vi "Test Depth.vi"() -> ()   [LabVIEW 2017]
doc: "Using the colors from the graph, make lines radiate from robot center in the direction of the camera. Depth values of 0 and maxInt are turned into NaNs, and that is the returned line of values."
uses:
  <vilib>/addons/RealSense/libRealSense3.lvlib
  <vilib>/Analysis/NI_AALPro.lvlib
  <vilib>/Analysis/NI_AALBase.lvlib
  <vilib>/vision/NI_Vision_Development_Module.lvlib
panel:
  in  "point offset":i32=15
  out "Array":T1(array[cluster])
  in  "side points":i32=15
  in  "Line #":i32(slide) scale=1.0..10.0
  out "Formula":string
  out "error":i32
  in  "Dialate":bool
  in  "File":bool
  in  "File #":i32(slide) scale=1.0..10.0
  out "Slope":dbl[][](graph)
  in  "Lines":i32=10
  out "Friltered":cluster{i32[], dbl[]}(graph)
  out "Image":T2(plugin-control)
  out "error out":errorcluster
  in  "stop":bool
  out "device count":i32
  # "All errors are #1, string is good"
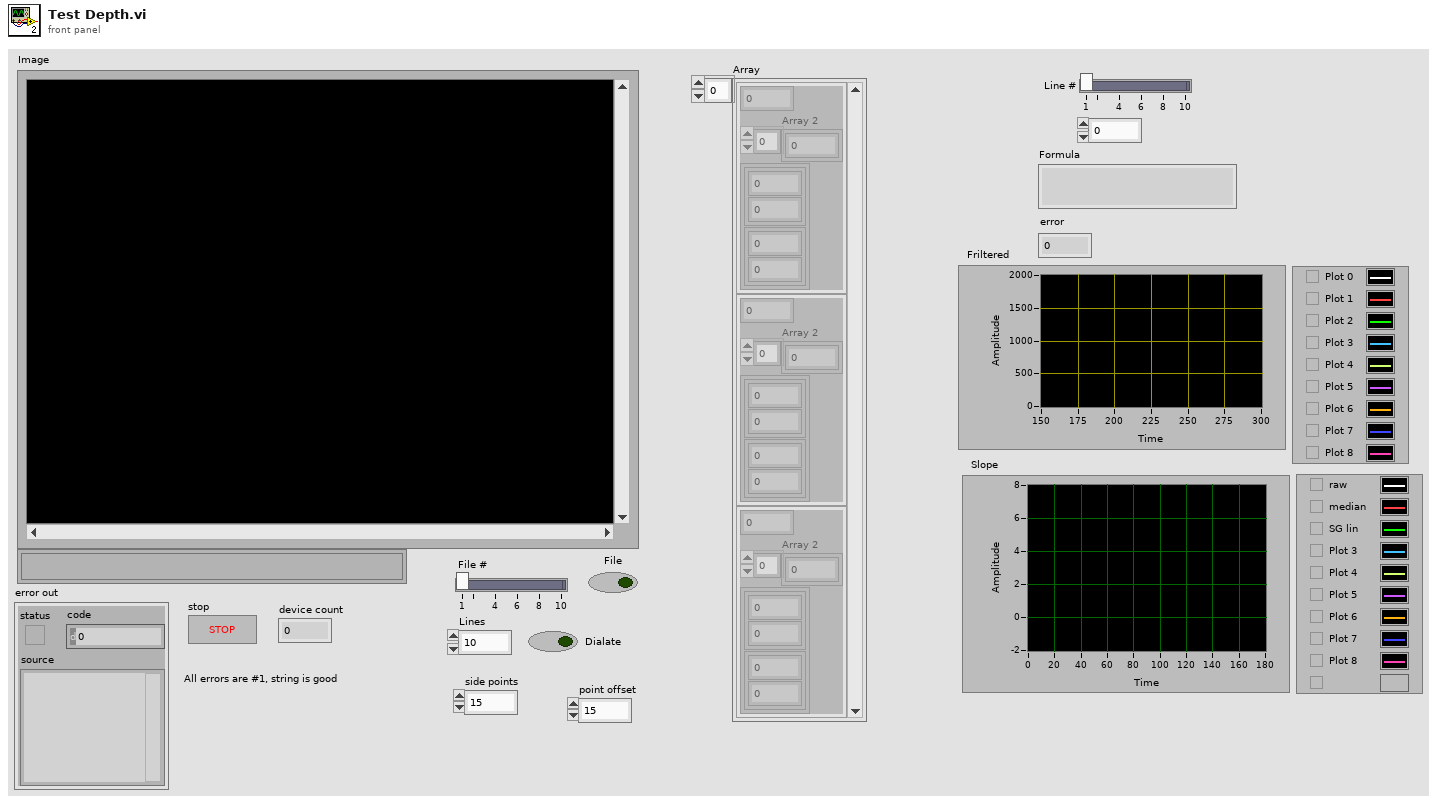
[diagram p1: front panel]
types:
  T1 = cluster{i32, "Array 2":i32[], cluster{cluster{dbl, dbl}, cluster{dbl, dbl}}}[]
  T2 = typedef "IMAQ Image.ctl" = refnum<image>
  T3 = typedef "Image Type" = u32
  T4 = cluster{"width":i32, "height":i32, "ppx":sgl, "ppy":sgl, "fx":sgl, "fy":sgl, "model":u32, "coeffs[0]":sgl, "coeffs[1]":sgl, "coeffs[2]":sgl, "coeffs[3]":sgl, "coeffs[4]":sgl}
  T5 = cluster{"Left":i32, "Top":i32, "Right":i32, "Bottom":i32}
  T6 = enum16{"Linear", "Polynomial", "Exponential", "Power"}
  T7 = cluster{i32, "Array 2":i32[], cluster{cluster{dbl, dbl}, cluster{dbl, dbl}}}
  T8 = cluster{"filtered indices":i32[], "filtered values":dbl[]}
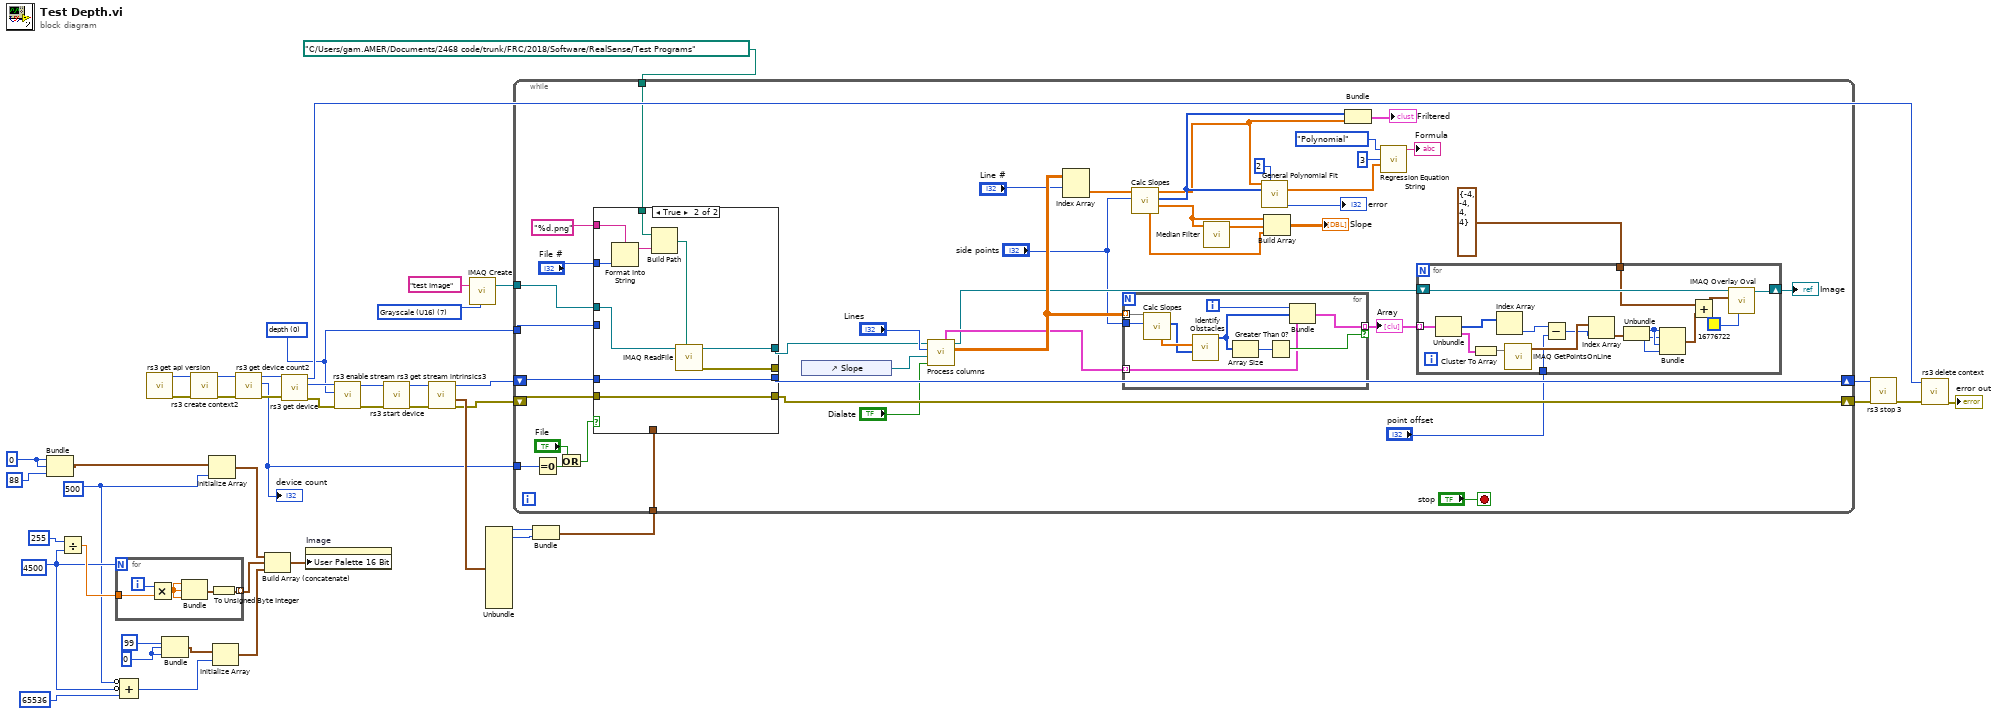
[diagram p0: block diagram]
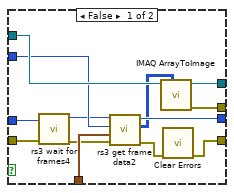
[diagram p2: hidden frame]
diagram:
  w3 = 4500
  w15 = u8 0
  w2 = 500
  w8 = u8 0
  w18 = u16 0 items=["depth", "color", "inf 1", "inf 2"] ("stream type")
  w20 = T3 7 items=["Grayscale (U8)", "Grayscale (I16)", "Grayscale (SGL)", "Complex (CSG)", "RGB (U32)", "HSL (U32)", "RGB (U64)", "Grayscale (U16)"] ("Image Type")
  n1 = Bundle(w8, w8, u8 88) -> (w16:cluster{u8, u8, u8})  [unwired: 1 in]
  n2 = Divide(x=u8 255, y=w3) -> (x/y=w6:dbl)
  n3 = for {
    N: w3 -> [_]
    tunnel: [w47] -> w10 mode=indexing
    tunnel: w6 -> [w46]
    i -> [w50]
    n4 = Multiply(x=w50, y=w46) -> (x*y=w49:dbl)
    n5 = Bundle(w49, w49, w49) -> (w48:cluster{dbl, dbl, dbl})  [unwired: 1 in]
    n6 = To Unsigned Byte Integer(number=w48) -> (unsigned 8bit integer=w47:cluster{u8, u8, u8})
  }
  n7 = Compound Arithmetic op=unknown(invert w2, invert w3, 65536) -> (w1:i32)
  n8 = call <vilib>:"rs3 get api version.vi"() -> ("error out"=w34:errorcluster, "version"=w45:i32)  [unwired: 10 in]
  n9 = Bundle(u8 99, w15, w15) -> (w13:cluster{u8, u8, u8})  [unwired: 1 in]
  n10 = call <vilib>:"rs3 create context2.vi"("error in (no error)"=w34, "version"=w45) -> ("error out"=w33:errorcluster, "context"=w44:u32)  [unwired: 8 in]
  n11 = Initialize Array(w16, w2) -> (w11:cluster{u8, u8, u8}[])
  n12 = Initialize Array(w13, w1) -> (w12:cluster{u8, u8, u8}[])
  n13 = call <vilib>:"rs3 get device count2.vi"("error in"=w33, "context"=w44) -> ("error out"=w32:errorcluster, "count"=w23:i32, "context"=w43:u32)  [unwired: 7 in]
  "device count" <- w23
  n14 = Build Array (concatenate)(w11, w10, w12) -> (w9:cluster{u8, u8, u8}[])
  n15 = call <vilib>:"rs3 get device.vi"("error in"=w32, "context"=w43) -> ("error out"=w31:errorcluster, "device"=w42:u32, "context"=w35:u64)  [unwired: 7 in]
  n16 = property on="Image" class="ImageControl"("User Palette 16 Bit"=w9) -> ()  [unwired: 2 in, 2 out]
  n17 = call <vilib>:"rs3 enable stream.vi"("error in"=w31, "stream type"=w18, "device"=w42) -> ("error out"=w30:errorcluster, "device"=w41:u32)  [unwired: 7 in]
  n18 = call <vilib>:"rs3 start device.vi"("error in"=w30, "device"=w41) -> ("error out"=w29:errorcluster, "device"=w40:u64)  [unwired: 8 in]
  n19 = call <vilib>:"rs3 get stream intrinsics3.vi"("error in (no error)"=w29, "device in"=w40) -> ("error out"=w28:errorcluster, "intrin out"=w38:T4, "device out"=w39:u64)  [unwired: 7 in]
  n20 = call "IMAQ Create"("Image Name"="test Image", "Image Type"=w20) -> ("New Image"=w19:T2)  [unwired: 3 in, 1 out]
  n21 = Unbundle(w38) -> ("width"=w26:i32, "height"=w25:i32)  [unwired: 10 out]
  n22 = Bundle("width"=w26, "height"=w25) -> (w24:cluster{"width":i32, "height":i32})  [unwired: 1 in]
  n23 = while {
    tunnel: w24 -> [w88]
    tunnel: w23 -> [w77]
    tunnel: w19 -> [w87]
    tunnel: w18 -> [w86]
    shift-right: [w91] -> w37
    shift-left: w39 -> [w92]
    shift-right: [w89] -> w27
    shift-left: w28 -> [w90]
    tunnel: path "C:/Users/gam.AMER/Documents/2468 code/trunk/FRC/2018/Software/RealSense/Test Programs" ("File Path") -> [w82]
    stop <- "stop" stop-if-true
    n24 = Equal To 0?(x=w77) -> (x = 0?=w79:bool)
    n25 = Or(x="File", y=w79) -> (x .or. y?=w76:bool)
    n26 = case shown="True" w76 {
      tunnel: w92 -> [w122 w132]
      tunnel: [w121 w132] -> w91
      tunnel: w90 -> [w120 w131]
      tunnel: [w119 w131] -> w89
      tunnel: w88 -> [w118 _]
      tunnel: w87 -> [w117 w130]
      tunnel: w86 -> [w116 _]
      tunnel: [w111 w129] -> w83
      tunnel: [w110 w123] -> _
      tunnel: w82 -> [_ w128]
      tunnel: "File #" -> [_ w126]
      tunnel: "%d.png" ("format string") -> [_ w124]
      frame False {
        n27 = call <vilib>:"rs3 wait for frames4.vi"("error in (no error)"=w120, "device in"=w122) -> ("error out"=w115:errorcluster, "device out"=w114:u64)  [unwired: 8 in]
        n28 = call <vilib>:"rs3 get frame data2.vi"("error in (no error)"=w115, "size"=w118, "stream type"=w116, "device in"=w114) -> ("error out"=w113:errorcluster, "2D Depth Output"=w112:u16[][], "device out"=w121:u64)  [unwired: 4 in, 1 out]
        n29 = call "IMAQ ArrayToImage"("Image Pixels (U16)"=w112, "Image"=w117) -> ("error out"=w110:errorcluster, "Image Out"=w111:T2)  [unwired: 8 in]
        n30 = call <vilib>:"Clear Errors.vi"("error in (no error)"=w113) -> ("error out"=w119:errorcluster)  [unwired: 5 in, 1 out]
      }
      frame True {
        n31 = Format Into String(format string=w124, w126) -> (resulting string=w125:string)  [unwired: 2 in, 1 out]
        n32 = Build Path(base path=w128, name or relative path=w125) -> (appended path=w127:path)
        n33 = call "IMAQ ReadFile"("File Path"=w127, "Image"=w130) -> ("error out"=w123:errorcluster, "Image Out"=w129:T2)  [unwired: 5 in, 3 out]
      }
    }
    n34 = control-ref of="Slope"() -> (w64:refnum<vi>)
    n35 = call "Process columns.vi"("Dialate"="Dialate", "WaveformGraph in"=w64, "Lines"="Lines", "Image Out"=w83) -> ("Filtered X"=w59:dbl[][], "Refnum out"=w55:T2, "Points"=w57:cluster{cluster{dbl, dbl}, cluster{dbl, dbl}}[])  [unwired: 4 in, 1 out]
    n36 = Index Array(array=w59, index (row)="Line #") -> (element=w68:dbl[])  [unwired: 1 in]
    n37 = for {
      tunnel: w59 -> [w142] mode=indexing
      tunnel: "side points" -> [w141]
      tunnel: [w137] -> w56 mode=indexing if=w135
      tunnel: w57 -> [w133] mode=indexing
      i -> [w138]
      n38 = call "Calc Slopes.vi"("side points"=w141, "Filtered X in"=w142) -> ("filtered indices"=w139:i32[], "Filtered Slopes"=w140:dbl[])  [unwired: 6 in, 2 out]
      n39 = call "Identify Obstacles.vi"("filtered indices"=w139, "Filtered Slopes"=w140) -> ("Array 2"=w134:i32[])  [unwired: 9 in]
      n40 = Array Size(array=w134) -> (size(s)=w136:i32)
      n41 = Greater Than 0?(x=w136) -> (x > 0?=w135:bool)
      n42 = Bundle(w138, "Array 2"=w134, w133) -> (w137:T7)  [unwired: 1 in]
    }
    "Array" <- w56
    n43 = call "Calc Slopes.vi"("side points"="side points", "Filtered X in"=w68) -> ("slopes"=w61:dbl[], "filtered indices"=w67:i32[], "filtered values"=w66:dbl[], "Filtered Slopes"=w60:dbl[])  [unwired: 6 in]
    n44 = call <vilib>:"Median Filter.vi"("X"=w61) -> ("Filtered X"=w63:dbl[])  [unwired: 9 in, 1 out]
    n45 = call <vilib>:"General Polynomial Fit.vi"("Y"=w66, "polynomial order"=2, "X"=w67) -> ("Polynomial Coefficients"=w72:dbl[], "error"=→"error":i32)  [unwired: 9 in, 2 out]
    n46 = Build Array(w61, w63, w60) -> (→"Slope":dbl[][])
    n47 = Bundle("filtered indices"=w67, "filtered values"=w66) -> (→"Friltered":T8)  [unwired: 1 in]
    n48 = call "Regression Equation String.vi"("coefficients"=w72, "precision"=3, "fit type"=T6."Polynomial") -> ("Formula"=→"Formula":string)  [unwired: 8 in]
    n49 = for {
      tunnel: w56 -> [w109] mode=indexing
      shift-right: [w107] -> w54
      shift-left: w55 -> [w108]
      tunnel: T5 {"Left"=-4, "Top"=-4, "Right"=4, "Bottom"=4} ("Bounding Rectangle") -> [w102]
      tunnel: "point offset" -> [w93]
      n50 = Unbundle(w109) -> ("Array 2"=w103:i32[], w106:cluster{cluster{dbl, dbl}, cluster{dbl, dbl}})  [unwired: 1 out]
      n51 = Cluster To Array(cluster=w106) -> (array=w105:cluster{dbl, dbl}[])
      n52 = Index Array(array=w103) -> (element=w95:i32)  [unwired: 1 in]
      n53 = call "IMAQ GetPointsOnLine"("Endpoints"=w105) -> ("Points of the Line"=w104:cluster{"X":i32, "Y":i32}[])  [unwired: 1 in, 2 out]
      n54 = Subtract(x=w95, y=w93) -> (x-y=w94:i32)
      n55 = Index Array(array=w104, index=w94) -> (element=w101:cluster{"X":i32, "Y":i32})
      n56 = Unbundle(w101) -> ("X"=w100:i32, "Y"=w99:i32)
      n57 = Bundle("X"=w100, "Y"=w99, "X"=w100, "Y"=w99) -> (w98:cluster{"X":i32, "Y":i32, "X":i32, "Y":i32})  [unwired: 1 in]
      n58 = Add(x=w102, y=w98) -> (x+y=w97:cluster{i32, i32, i32, i32})
      n59 = call "IMAQ Overlay Oval"("Color"=u32 16776722, "Bounding Rectangle"=w97, "Image"=w108) -> ("Image Out"=w107:T2)  [unwired: 7 in, 1 out]
    }
    "Image" <- w54
  }
  n60 = call <vilib>:"rs3 stop 3.vi"("error in (no error)"=w27, "device"=w37) -> ("error out"=w36:errorcluster)  [unwired: 8 in, 1 out]
  n61 = call <vilib>:"rs3 delete context.vi"("error in (no error)"=w36, "context"=w35) -> ("error out"=→"error out":errorcluster)  [unwired: 9 in]
